vi "Save Load Settings.vi"(8 "error in":errorcluster, 10 "Dashboard Data (in)":T1={"Drive PID - Low"={"D"=0.0, "F"=0.0, "RR"=0.0, "IZ"=0.0, "P"=0.0, "I"=0.0}, "Drive PID - High"={"D"=0.0, "F"=0.0, "RR"=0.0, "IZ"=0.0, "P"=0.0, "I"=0.0}, "Vision Settings"={"LED Color"={"Hue"={107.81818389892578, 139.81818389892578}, "Sat"={176.07142857142858, 255.0}, "Val"={40.53571428571429, 255.0}}}, "Robot Name"="", "Winch Out"=0.0, "Winch In"=0.0} {"Vision Settings"."LED Color"."Hue" scale=0.0..255.0 scale format="%#_3g"}, 11 "Save Load Info":T3) -> (0 "error out":errorcluster, 2 "Dashboard Data (out)":T1={"Drive PID - Low"={"D"=0.0, "F"=0.0, "RR"=0.0, "IZ"=0.0, "P"=0.0, "I"=0.0}, "Drive PID - High"={"D"=0.0, "F"=0.0, "RR"=0.0, "IZ"=0.0, "P"=0.0, "I"=0.0}, "Vision Settings"={"LED Color"={"Hue"={107.81818389892578, 139.81818389892578}, "Sat"={176.07142857142858, 255.0}, "Val"={40.53571428571429, 255.0}}}, "Robot Name"="", "Winch Out"=0.0, "Winch In"=0.0} {"Vision Settings"."LED Color"."Hue" scale=0.0..255.0 scale format="%#_3g"}, 3 "Save Load Info (out)":T3)   [LabVIEW 2016]
uses:
  Load Save Info.ctl
  <vilib>/Utility/config.llb/Config Data RefNum.ctl
  Dashboard Data.ctl
  PID Settings.ctl
  <vilib>/Rock Robotics/Network Tables/NT Write Boolean.vi
  <vilib>/Utility/config.llb/NI_LVConfig.lvlib
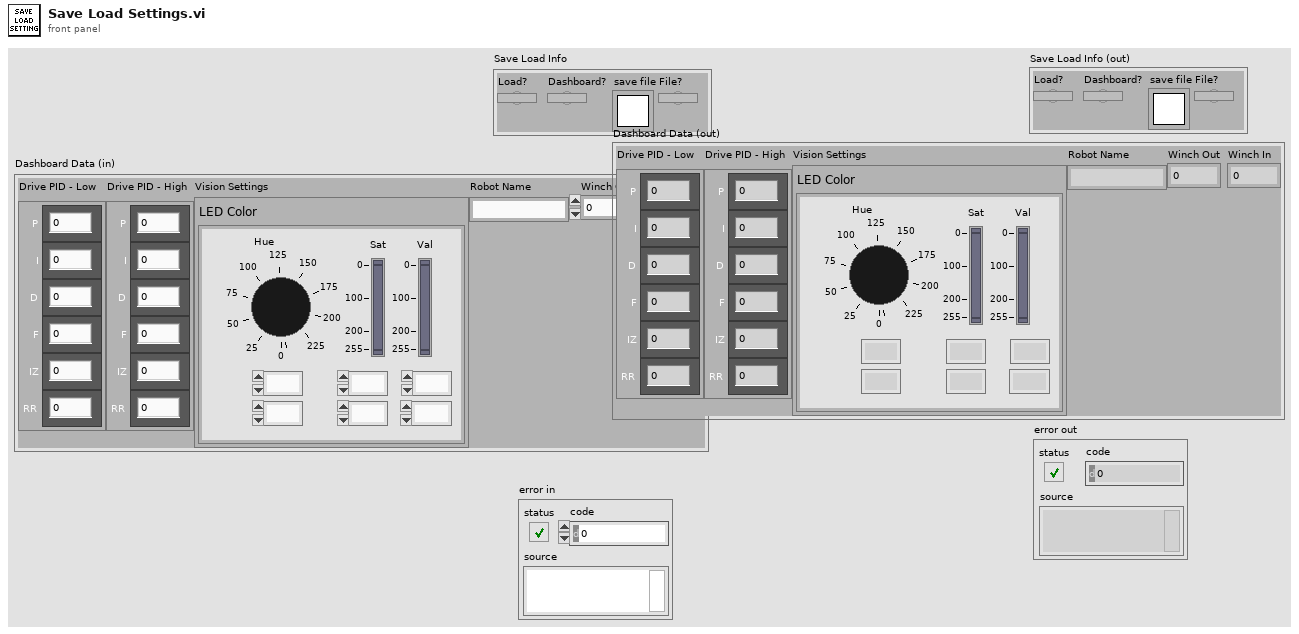
[diagram p1: front panel]
types:
  T1 = typedef "Dashboard Data.ctl" = cluster{"Drive PID - Low":T2, "Drive PID - High":T2, "Vision Settings":cluster{"LED Color":cluster{"Hue":cluster{dbl, dbl}, "Sat":cluster{dbl, dbl}, "Val":cluster{dbl, dbl}}}, "Robot Name":string, "Winch Out":dbl, "Winch In":dbl}
  T2 = typedef "PID Settings.ctl" = cluster{"D":dbl, "F":dbl, "RR":dbl, "IZ":dbl, "P":dbl, "I":dbl}
  T3 = typedef "Load Save Info.ctl" = cluster{"Load?":bool, "Dashboard?":bool, "save file":T4, "File?":bool}
  T4 = typedef "NI_LVConfig.lvlib/Config Data RefNum.ctl" = refnum<k1>
  T5 = cluster{"LED Color":cluster{"Hue":cluster{dbl, dbl}, "Sat":cluster{dbl, dbl}, "Val":cluster{dbl, dbl}}}
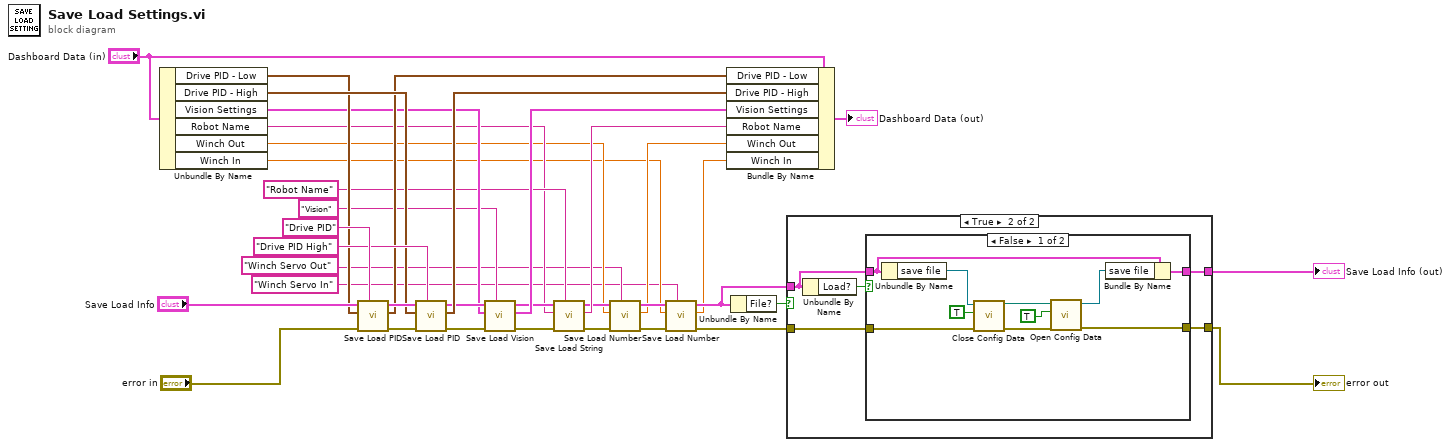
[diagram p0: block diagram]
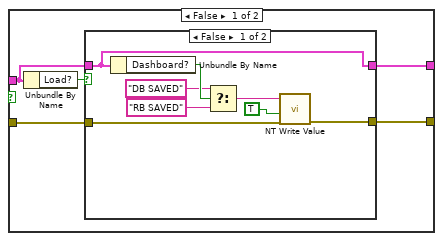
[diagram p2: hidden frame]
diagram:
  n1 = Unbundle By Name("Dashboard Data (in)") -> ("Drive PID - Low"=w27:T2, "Drive PID - High"=w28:T2, "Vision Settings"=w19:T5, "Robot Name"=w14:string, "Winch Out"=w6:dbl, "Winch In"=w4:dbl)
  n2 = call "Save Load PID.vi"("Name"="Drive PID", "error in"="error in", "PID (in)"=w27, "Save Load Info (in)"="Save Load Info") -> ("error out"=w31:errorcluster, "PID (out)"=w25:T2, "Save Load Info (out)"=w30:T3)  [unwired: 5 in]
  n3 = call "Save Load PID.vi"("Name"="Drive PID High", "error in"=w31, "PID (in)"=w28, "Save Load Info (in)"=w30) -> ("error out"=w21:errorcluster, "PID (out)"=w24:T2, "Save Load Info (out)"=w22:T3)  [unwired: 5 in]
  n4 = call "Save Load Vision.vi"("Name"="Vision", "error in"=w21, "Vision Settings (in)"=w19, "Save Load Info (in)"=w22) -> ("error out"=w15:errorcluster, "Vision Settings (out)"=w20:T5, "Save Load Info (out)"=w17:T3)  [unwired: 5 in]
  n5 = call "Save Load String.vi"("Name"="Robot Name", "error in"=w15, "String (in)"=w14, "Save Load Info (in)"=w17) -> ("error out"=w12:errorcluster, "String (out)"=w13:string, "Save Load Info (out)"=w8:T3)  [unwired: 5 in]
  n6 = call "Save Load Number.vi"("Name"="Winch Servo Out", "error in"=w12, "Num (in)"=w6, "Save Load Info (in)"=w8) -> ("error out"=w10:errorcluster, "Num (out)"=w5:dbl, "Save Load Info (out)"=w11:T3)  [unwired: 5 in]
  n7 = call "Save Load Number.vi"("Name"="Winch Servo In", "error in"=w10, "Num (in)"=w4, "Save Load Info (in)"=w11) -> ("error out"=w9:errorcluster, "Num (out)"=w3:dbl, "Save Load Info (out)"=w7:T3)  [unwired: 5 in]
  n8 = Bundle By Name(cluster="Dashboard Data (in)", "Drive PID - Low"=w25, "Drive PID - High"=w24, "Vision Settings"=w20, "Robot Name"=w13, "Winch Out"=w5, "Winch In"=w3) -> (→"Dashboard Data (out)":T1)
  n9 = Unbundle By Name(w7) -> ("File?"=w34:bool)
  n10 = case shown="True" w34 {
    tunnel: w9 -> [w38 w56]
    tunnel: w7 -> [w40 w55]
    tunnel: [w41 w54] -> w32
    tunnel: [w39 w53] -> w33
    frame False {
      n11 = Unbundle By Name(w40) -> ("Load?"=w42:bool)
      n12 = case shown="False" w42 {
        tunnel: [w44 w52] -> w41
        tunnel: w40 -> [w44 w52]
        tunnel: [w46 w51] -> w39
        tunnel: w38 -> [w45 w51]
        frame False {
          n13 = Unbundle By Name(w44) -> ("Dashboard?"=w50:bool)
          n14 = Select(t="DB SAVED" ("Name"), s=w50, f="RB SAVED" ("Name")) -> (s? t:f=w47:string)
          n15 = call-poly <vilib>:"NT Write Value.vi"("error in"=w45, "Boolean"=TRUE, "Name"=w47) -> ("error out"=w46:errorcluster)  [unwired: 8 in]
        }
        frame True {
        }
      }
    }
    frame True {
      n16 = Unbundle By Name(w55) -> ("Load?"=w57:bool)
      n17 = case shown="False" w57 {
        tunnel: w56 -> [w62 w68]
        tunnel: w55 -> [w60 w69]
        tunnel: [w61 w68] -> w53
        tunnel: [w58 w69] -> w54
        frame False {
          n18 = Unbundle By Name(w60) -> ("save file"=w63:T4)
          n19 = call <vilib>:"Close Config Data.vi"("error in (no error)"=w62, "write file if changed (T)"=TRUE, "refnum"=w63) -> ("error out"=w66:errorcluster, "file path"=w64:path)  [unwired: 7 in]
          n20 = call <vilib>:"Open Config Data.vi"("error in (no error)"=w66, "create file if necessary (T)"=TRUE, "configuration file path"=w64) -> ("error out"=w61:errorcluster, "refnum"=w59:T4)  [unwired: 6 in, 1 out]
          n21 = Bundle By Name(cluster=w60, "save file"=w59) -> (w58:T3)
        }
        frame True {
        }
      }
    }
  }
  "Save Load Info (out)" <- w32
  "error out" <- w33
